vi "RedistributeArmAbsolutePose.vi"(1 "DesiredPointSpacing (in)":dbl, 2 "OriginalPoints":T1[](array[typedef])) -> (0 "RedistributedPoints":T1[](array[typedef]))   [LabVIEW 2018]
uses:
  TypeDefs/ArmAbsolutePosition.ctl
  ArgosLib/ArgosLib.lvlib
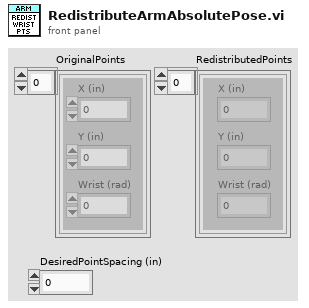
[diagram p1: front panel]
types:
  T1 = typedef "ArmAbsolutePosition.ctl" = cluster{"X (in)":dbl, "Y (in)":dbl, "Wrist (rad)":dbl}
  T2 = typedef "ArgosLib.lvlib/Point2D.ctl" = cluster{"X (in)":dbl, "Y (in)":dbl}
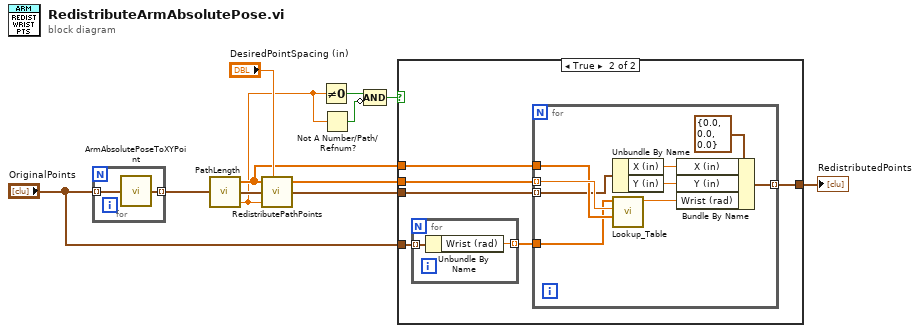
[diagram p0: block diagram]
diagram:
  n1 = for {
    tunnel: "OriginalPoints" -> [w14] mode=indexing
    tunnel: [w13] -> w10 mode=indexing
    n2 = call "ArmAbsolutePoseToXYPoint.vi"("ArmAbsolutePose"=w14) -> ("2DPoint"=w13:T2)
  }
  n3 = call "PathLength.vi"("PathIn"=w10) -> ("Path Length"=w1:dbl, "PathOut"=w12:T2[], "IndexedPathLength"=w3:dbl[])  [unwired: 2 in]
  n4 = call "RedistributePathPoints.vi"("IndexedPathLength"=w3, "Desired Point Spacing (in)"="DesiredPointSpacing (in)", "PathIn"=w12, "Path Length (in)"=w1) -> ("IndexedPathLengthOut"=w4:dbl[], "PathOut"=w2:T2[])  [unwired: 2 in]
  n5 = Not Equal To 0?(x=w1) -> (x != 0?=w9:bool)
  n6 = Not A Number/Path/Refnum?(number/path/refnum=w1) -> (NaN/Path/Refnum?=w8:bool)
  n7 = Compound Arithmetic op=AND(w9, invert w8) -> (w7:bool)
  n8 = case shown="True" w7 {
    tunnel: "OriginalPoints" -> [w15 w21]
    tunnel: [w15 w16] -> w5
    tunnel: w4 -> [_ w20]
    tunnel: w3 -> [_ w19]
    tunnel: w2 -> [_ w17]
    frame False {
    }
    frame True {
      n9 = for {
        tunnel: w21 -> [w23] mode=indexing
        tunnel: [w22] -> w18 mode=indexing
        n10 = Unbundle By Name(w23) -> ("Wrist (rad)"=w22:dbl)
      }
      n11 = for {
        tunnel: w20 -> [w32] mode=indexing
        tunnel: w19 -> [w31]
        tunnel: w18 -> [w30]
        tunnel: w17 -> [w26] mode=indexing
        tunnel: [w28] -> w16 mode=indexing
        n12 = Unbundle By Name(w26) -> ("X (in)"=w25:dbl, "Y (in)"=w24:dbl)
        n13 = call "Lookup_Table.vi"("Y_Array"=w30, "x_in"=w32, "X_Array"=w31) -> ("y_out"=w27:dbl)  [unwired: 6 in]
        n14 = Bundle By Name(cluster=T1 {"X (in)"=0.0, "Y (in)"=0.0, "Wrist (rad)"=0.0} ("ArmAbsolutePose"), "X (in)"=w25, "Y (in)"=w24, "Wrist (rad)"=w27) -> (w28:T1)
      }
    }
  }
  "RedistributedPoints" <- w5
